vi "CAN Set Value.vi"(7 "BufferLength":u32, 9 "Buffer":u32, 10 "Parameter":u8, 11 "Channel":u16) -> (1 "Buffer out":u32, 3 "function return":u32)   [LabVIEW 2020, in "PCANBasic.lvlib"]
doc: "TPCANStatus __stdcall CAN_SetValue(\n TPCANHandle Channel,\n TPCANParameter Parameter,\n void* Buffer,\n DWORD BufferLength);"
uses:
  <userlib>/PCANBasic/PCANBasic.lvlib
  <userlib>/PCANBasic/PCANBasic.dll
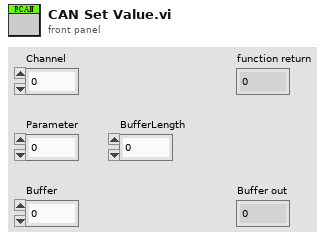
[diagram p1: front panel]
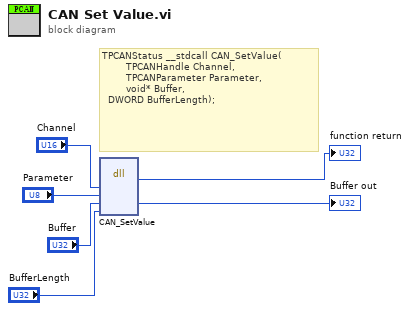
[diagram p0: block diagram]
diagram:
  # "TPCANStatus __stdcall CAN_SetValue(\n        TPCANHandle Channel,\n        TPCANParameter Parameter,\n        void* Buffer,\n\t\tDWORD BufferLength);"
  n1 = dll-call lib="D:/Program Files (x86)/National Instruments/LabVIEW 2020/user.lib/PCANBasic/PCANBasic.*" fn="CAN_SetValue"("Channel"="Channel", "Parameter"="Parameter", "Buffer"="Buffer", "BufferLength"="BufferLength") -> (→"function return":u32, "Buffer"=→"Buffer out":u32)  [unwired: 6 in, 2 out]
